vi "LSMcontroller_v61_updatedROIselection.vi"() -> ()   [LabVIEW 2015] (continued)
                            n1350 = call "stoperaseCI.vi"() -> ()  [unwired: 12 in]
                            n1351 = call "stoperaseDO_img.vi"() -> ()  [unwired: 12 in]
                            n1352 = call "stoperaseAO_img.vi"() -> ()  [unwired: 12 in]
                            n1353 = call "stoperaseAI_img.vi"() -> ()  [unwired: 12 in]
                          }
                          frame #7 {
                            w3778 = T22 2 items=["no dialog", "OK message", "continue or stop message", "OK message + warnings", "continue/stop + warnings"] ("type of dialog (OK msg:1)")
                            n1354 = call "displayerrors.vi"() -> ("error IO"=w3779:errorcluster)
                            n1355 = call <vilib>:"General Error Handler.vi"("type of dialog (OK msg:1)"=w3778, "error in (no error)"=w3779) -> ("error out"=w3777:errorcluster)  [unwired: 9 in, 4 out]
                            n1356 = call <vilib>:"Clear Errors.vi"("error in (no error)"=w3777) -> ("error out"=w3776:errorcluster)  [unwired: 5 in, 1 out]
                            n1357 = call "seterrors.vi"("error IO"=w3776) -> ()
                          }
                          frame #8 {
                            w3789 = FALSE ("Value (Signaling)")
                            n1358 = local read "save\ndata"() -> (w3784:bool)
                            n1359 = call "2pparameters.vi"("command"="get") -> ("params out"=w3782:T11)  [unwired: 1 in]
                            n1360 = Unbundle By Name(w3782) -> ("auto OD"=w3780:bool)
                            n1361 = case shown="True" w3784 {
                              tunnel: w3783 -> [_ w3796]
                              frame False {
                              }
                              frame True {
                                n1362 = local read "filename prefix"() -> (w3797:string)
                                n1363 = call "closebinaryfiles.vi"() -> ()  [unwired: 12 in]
                                n1364 = local read "data dir"() -> (w3798:path)
                                n1365 = call "saveparams.vi"("timestamp"=w3796, "filename prefix in"=w3797, "data dir in"=w3798) -> ()  [unwired: 1 in]
                              }
                            }
                            n1366 = case shown="True" w3780 {
                              frame False {
                              }
                              frame True {
                                n1367 = call "configuration.vi"("command"="get") -> ("config out"=w3792:T12)  [unwired: 2 in, 1 out]
                                n1368 = call "2pparameters.vi"("command"="get") -> ("params out"=w3795:T11)  [unwired: 1 in]
                                n1369 = Unbundle By Name(w3792) -> ("point OD"=w3790:u16)
                                n1370 = Unbundle By Name(w3795) -> ("ODfilt"=w3791:u16)
                                n1371 = call "filterwheelcontrol_nothorlabslib.vi"("Current OD filt"=w3790, "New ODfilt"=w3791) -> ()  [unwired: 1 in]
                              }
                            }
                            n1372 = call "reset AO_DO_v3.vi"() -> ()  [unwired: 12 in]
                            n1373 = property on="Start" class="Bool (strict)"("Val(Sgnl)"=w3789) -> ()  [unwired: 2 in, 2 out]
                            n1374 = property on="Start" class="Bool (strict)"("Visible"=TRUE, "DisabledEnum"=T7."Enabled" ("Disabled")) -> ()  [unwired: 2 in, 2 out]
                            n1375 = property on="Stop" class="Bool (strict)"("Val(Sgnl)"=w3789) -> ()  [unwired: 2 in, 2 out]
                            n1376 = property on="Stop" class="Bool (strict)"("Visible"=FALSE, "DisabledEnum"=T7."Disabled" ("Disabled")) -> ()  [unwired: 2 in, 2 out]
                          }
                        }
                      }
                      frame "Line" {
                      }
                      frame "Resonant Ellipse", "freeform contour", "Fill Ellipse" {
                        n1377 = stacked-sequence {
                          seq-local: [w3813 _ _ _ _ _ _ _ _ _ _] -> [_ _ w4658 _ _ w4671 w4738 _ _ w5098 _]
                          seq-local: [w3812 _ _ _ _ _ _ _ _ _ _] -> [_ _ _ _ _ _ _ _ w4785 _ _]
                          seq-local: [w3811 _ _ _ _ _ _ _ _ _ _] -> [_ _ _ _ _ _ _ _ w4784 _ _]
                          seq-local: [w3810 _ _ _ _ _ _ _ _ _ _] -> [_ _ _ _ _ _ _ _ w4787 _ _]
                          seq-local: [w3809 _ _ _ _ _ _ _ _ _ _] -> [_ _ _ _ _ _ _ _ w4783 _ _]
                          seq-local: [w3808 _ _ _ _ _ _ _ _ _ _] -> [_ _ _ _ _ _ _ _ w4782 _ _]
                          seq-local: [w3807 _ _ _ _ _ _ _ _ _ _] -> [_ _ _ _ _ _ _ _ w4786 _ _]
                          seq-local: [w3806 _ _ _ _ _ _ _ _ _ _] -> [_ _ _ _ _ _ _ _ w4781 _ _]
                          seq-local: [w3805 _ _ _ _ _ _ _ _ _ _] -> [_ _ _ _ _ _ _ _ w4780 _ _]
                          seq-local: [w3804 _ _ _ _ _ _ _ _ _ _] -> [_ _ _ _ _ _ _ _ w4775 _ _]
                          seq-local: [w3803 _ _ _ _ _ _ _ _ _ _] -> [_ _ _ _ _ _ _ _ w4774 _ _]
                          seq-local: [w3802 _ _ _ _ _ _ _ _ _ _] -> [_ _ _ _ _ _ _ _ w4779 _ _]
                          seq-local: [w3801 _ _ _ _ _ _ _ _ _ _] -> [_ _ _ _ _ _ _ _ w4778 _ _]
                          seq-local: [w3800 _ _ _ _ _ _ _ _ _ _] -> [_ _ _ _ _ _ _ _ w4777 _ _]
                          seq-local: [w3799 _ _ _ _ _ _ _ _ _ _] -> [_ _ _ _ _ _ _ _ w4776 _ _]
                          frame #0 {
                            n1378 = local read "save\ndata"() -> (w3814:bool)
                            n1379 = Get Date/Time In Seconds() -> (seconds since 1Jan1904=w3815:timestamp)
                            n1380 = case shown="False" w3814 {
                              tunnel: w3815 -> [w3816 w3818]
                              tunnel: [w3816 w3817] -> w3813
                              frame False {
                              }
                              frame True {
                                n1381 = call "createdatafolder.vi"("timestamp in"=w3818) -> ("current data path"=w3819:path, "timestamp out"=w3817:timestamp)
                                n1382 = local write "data dir"(w3819) -> ()
                              }
                            }
                            n1383 = stacked-sequence {
                              tunnel: w3813 -> [w3825 _ _ _ _ _ _ _ _]
                              tunnel: [_ _ _ _ _ _ w3963 _ _] -> w3812
                              tunnel: [_ _ _ _ _ _ w3962 _ _] -> w3811
                              tunnel: [_ _ _ _ _ _ w3961 _ _] -> w3810
                              tunnel: [_ _ _ _ _ _ w3960 _ _] -> w3809
                              tunnel: [_ _ _ _ _ _ w3959 _ _] -> w3808
                              tunnel: [_ _ _ _ _ _ w3958 _ _] -> w3807
                              tunnel: [_ _ _ _ _ _ w3957 _ _] -> w3806
                              tunnel: [_ _ _ _ _ _ w3956 _ _] -> w3805
                              tunnel: [_ _ _ _ _ _ w3955 _ _] -> w3804
                              tunnel: [_ _ _ _ _ _ w3954 _ _] -> w3803
                              tunnel: [_ _ _ _ _ _ w3953 _ _] -> w3802
                              tunnel: [_ _ _ _ _ _ w3952 _ _] -> w3801
                              tunnel: [_ _ _ _ _ _ w3951 _ _] -> w3800
                              tunnel: [_ _ _ _ _ _ w3950 _ _] -> w3799
                              frame #0 {
                                n1384 = local write "graphtab"(T5."timetrace" ("graphtab")) -> ()
                                n1385 = local read "AI channels"() -> (w3829:i32[])
                                n1386 = local read "CI channels"() -> (w3830:i32[])
                                n1387 = property on="Stop" class="Bool (strict)"("Visible"=TRUE, "DisabledEnum"=T7."Enabled" ("Disabled")) -> ()  [unwired: 2 in, 2 out]
                                n1388 = property on="Start" class="Bool (strict)"("Visible"=FALSE, "DisabledEnum"=T7."Disabled and Grayed Out" ("Disabled")) -> ()  [unwired: 2 in, 2 out]
                                n1389 = Format Date/Time String(time format string (%c)="%Y%m%d", seconds (now)=w3825) -> (date/time string=w3824:string)  [unwired: 1 in]
                                n1390 = Format Date/Time String(time format string (%c)="%H%M%S", seconds (now)=w3825) -> (date/time string=w3823:string)  [unwired: 1 in]
                                n1391 = call "2pparameters.vi"("command"="get") -> ("params out"=w3832:T11)  [unwired: 1 in]
                                n1392 = Bundle By Name(cluster=w3832, "aAI"=w3829, "aCI"=w3830, "type"="Timetrace", "date"=w3824, "time"=w3823) -> (w3831:T11)
                                n1393 = call "X-array-databuffer.vi"("command"=enum16{"get", "set", "clear", "append"}."clear") -> ()  [unwired: 3 in, 2 out]
                                n1394 = call "Y-array-databuffer.vi"("command"=enum16{"get", "set", "clear", "append"}."clear") -> ()  [unwired: 3 in, 2 out]
                                n1395 = call "2pparameters.vi"("Params in"=w3831, "command"="set") -> ()  [unwired: 1 out]
                                n1396 = call "CH1-1D-temp.vi"("command"=enum16{"get", "set", "clear", "append"}."clear") -> ()  [unwired: 3 in, 2 out]
                                n1397 = call "CH2-1D-temp.vi"("command"=enum16{"get", "set", "clear", "append"}."clear") -> ()  [unwired: 3 in, 2 out]
                                n1398 = call "allAI-temp.vi"("command"=enum16{"get", "set", "clear", "append"}."clear") -> ()  [unwired: 3 in, 2 out]
                              }
                              frame #1 {
                                n1399 = call "configuration.vi"("command"="get") -> ("config out"=w3849:T12)  [unwired: 2 in, 1 out]
                                n1400 = Unbundle By Name(w3849) -> ("CI names"=w3850:string[], "AI names"=w3851:string[])
                                n1401 = call "2pparameters.vi"("command"="get") -> ("params out"=w3845:T11)  [unwired: 1 in]
                                n1402 = Unbundle By Name(w3845) -> ("aCI"=w3846:i32[], "aAI"=w3847:i32[])
                                n1403 = for {
                                tunnel: w3846 -> [w3861] mode=indexing
                                tunnel: w3850 -> [w3862]
                                tunnel: [w3860] -> w3852 mode=indexing
                                n1404 = Index Array(array=w3862, index=w3861) -> (element=w3860:string)
                                }
                                n1405 = for {
                                tunnel: w3847 -> [w3858] mode=indexing
                                tunnel: w3851 -> [w3859]
                                tunnel: [w3857] -> w3853 mode=indexing
                                n1406 = Index Array(array=w3859, index=w3858) -> (element=w3857:string)
                                }
                                n1407 = Build Array (concatenate)(w3852, w3853) -> (w3843:string[])
                                n1408 = for {
                                tunnel: w3843 -> [w3855] mode=indexing
                                tunnel: [w3854] -> w3842 mode=indexing
                                i -> [w3856]
                                n1409 = Bundle("String"=w3855, w3856) -> (w3854:cluster{"String":string, i32})  [unwired: 1 in]
                                }
                                n1410 = property on="graph1list" class="Ring (strict)"("StringsAndValues[]"=w3842) -> ()  [unwired: 2 in, 2 out]
                                n1411 = property on="graph2list" class="Ring (strict)"("StringsAndValues[]"=w3842) -> ()  [unwired: 2 in, 2 out]
                              }
                              frame #2 {
                                n1412 = call "2pparameters.vi"("command"="get") -> ("params out"=w3865:T11)  [unwired: 1 in]
                                n1413 = Unbundle By Name(w3865) -> ("auto OD"=w3863:bool, "autoshutter"=w3866:bool)
                                n1414 = case shown="True" w3863 {
                                frame False {
                                }
                                frame True {
                                n1415 = call "configuration.vi"("command"="get") -> ("config out"=w3869:T12)  [unwired: 2 in, 1 out]
                                n1416 = Unbundle By Name(w3869) -> ("contour OD"=w3870:u16)
                                n1417 = local read "ODfilt"() -> (w3867:u16)
                                n1418 = call "filterwheelcontrol_nothorlabslib.vi"("Current OD filt"=w3867, "New ODfilt"=w3870) -> ()  [unwired: 1 in]
                                }
                                }
                                n1419 = case shown="True" w3866 {
                                frame False {
                                }
                                frame True {
                                n1420 = call "shuttercontrol.vi"("command"="close") -> ()  [unwired: 1 in, 1 out]
                                }
                                }
                              }
                              frame #3 {
                                n1421 = local read "Vy-min draw"() -> (w3879:dbl)
                                n1422 = local read "Vy-max draw"() -> (w3878:dbl)
                                n1423 = local read "Vx-min draw"() -> (w3881:dbl)
                                n1424 = local read "Vx-max draw"() -> (w3880:dbl)
                                n1425 = local read "xpixels ref"() -> (w3877:i32)
                                n1426 = local read "ypixels ref"() -> (w3876:i32)
                                n1427 = local read "ROI Type"() -> (w3875:u16)
                                n1428 = local read "srateAODOtt"() -> (w3898:dbl)
                                n1429 = local read "# of frames"() -> (w3903:i32)
                                n1430 = local read "refreshtime"() -> (w3895:dbl)
                                n1431 = local read "Pel"() -> (w3874:dbl)
                                n1432 = local read "bin"() -> (w3901:dbl)
                                n1433 = local read "Override AI buffer"() -> (w3872:bool)
                                n1434 = local read "finite samples"() -> (w3910:bool)
                                n1435 = local read "srateAODOtt"() -> (w3897:dbl)
                                n1436 = local read "srateAODOtt"() -> (w3904:dbl)
                                n1437 = local read "continuous"() -> (w3909:bool)
                                n1438 = local read "Angle ref"() -> (w3882:dbl)
                                n1439 = local read "wavdet"() -> (w3911:bool)
                                n1440 = local read "Vx-ref"() -> (w3906:dbl)
                                n1441 = local read "Vy-ref"() -> (w3908:dbl)
                                n1442 = local read "avpp"() -> (w3907:i32)
                                n1443 = call "tt_timeandsamples.vi"("bin"=w3901, "refreshtime"=w3895, "srateAODOtt"=w3898, "tot#ofsamples"=w3903) -> ("refreshrate"=w3899:dbl, "refreshbuffer"=w3900:i32, "timetracecycles"=w3905:i32)  [unwired: 5 in]
                                n1444 = local read "bin"() -> (w3902:dbl)
                                n1445 = call "2pparameters.vi"("command"="get") -> ("params out"=w3914:T11)  [unwired: 1 in]
                                n1446 = Bundle By Name(cluster=w3914, "Drawing Mode"=w3875, "measpoints"=w3903, "tt_cycles"=w3905, "refreshbuffer"=w3900, "refreshrate"=w3899, "Vx-ref"=w3906, "Vy-ref"=w3908, "srate"=w3897, "finite"=w3910, "cont"=w3909, "wavdet"=w3911, "avpp"=w3907, "srateAODO"=w3904, "bufferAI"=w3900, "bin"=w3902, "Angle Img"=w3882, "Vxminref"=w3881, "Vxmaxref"=w3880, "Vyminref"=w3879, "Vymaxref"=w3878, "Xpixels Img"=w3877, "Ypixels Img"=w3876, "Pel"=w3874, "Vz-reset"=0.0, "AIoverride"=w3872) -> (w3912:T11)
                                n1447 = Reciprocal(x=w3899) -> (1/x=w3896:dbl)
                                n1448 = local write "refreshtime"(w3896) -> ()
                                n1449 = call "2pparameters.vi"("Params in"=w3912, "command"="set") -> ()  [unwired: 1 out]
                                n1450 = local read "Voltage Clamp"() -> (w3889:bool)
                                n1451 = local read "Current Clamp"() -> (w3890:bool)
                                n1452 = local read "Vholding (mV)"() -> (w3884:sgl)
                                n1453 = local read "CC_ICgain"() -> (w3888:dbl)
                                n1454 = local read "OCgain"() -> (w3885:sgl)
                                n1455 = local read "holdon"() -> (w3883:bool)
                                n1456 = call "patchparameters.vi"("command"="get") -> ("Params out"=w3892:T14)  [unwired: 1 in]
                                n1457 = Bundle By Name(cluster=w3892, "VC"=w3889, "CC"=w3890, "CC_icg (pA/mv)"=w3888, "VC_icg (mV/mV)"=10.0, "OCG (mV/pA)"=w3885, "OVG (mV/mV)"=0.1, "Vhold (mV)"=w3884, "holdon"=w3883) -> (w3891:T14)
                                n1458 = call "patchparameters.vi"("Params in"=w3891, "command"="set") -> ()  [unwired: 1 out]
                              }
                              frame #4 {
                                n1459 = call "2pparameters.vi"("command"="get") -> ("params out"=w3930:T11)  [unwired: 1 in]
                                n1460 = Unbundle By Name(w3930) -> ("srateAODO"=w3931:sgl, "Angle Img"=w3932:dbl, "Angle draw"=w3933:dbl, "Vxmaxref"=w3934:dbl, "Vxminref"=w3935:dbl, "Xpixels Img"=w3936:i32, "Ypixels Img"=w3937:i32, "Vymaxref"=w3938:dbl, "Vxminref"=w3939:dbl, "Drawing Mode"=w3940:u16, "Pel"=w3941:sgl)
                                n1461 = Add(x=w3932, y=w3933) -> (x+y=w3916:dbl)
                                n1462 = call "ROI-databuffer.vi"("command"=enum16{"get", "set", "clear", "append"}."get") -> ("array out"=w3924:cluster{"x":sgl, "y":sgl}[])  [unwired: 4 in]
                                n1463 = call "ScanningWaveform_v4.vi"("Vy-min"=w3939, "Vy-max"=w3938, "yPixels/tPixels"=w3937, "xPixels/rPixels"=w3936, "Vx-min"=w3935, "Vx-max"=w3934, "Drawing Mode"=w3940, "Angle"=w3916, "AOrate"=w3931, "Points"=w3924, "points in ellipse"=w3941) -> ("numPixels"=w3917:dbl, "Y-WaveArray"=w3918:dbl[], "P"=w3923:dbl, "X-WaveArray"=w3919:dbl[])  [unwired: 5 in]
                                n1464 = call "Y-array-databuffer.vi"("array in"=w3918, "command"=enum16{"get", "set", "clear", "append"}."set") -> ()  [unwired: 2 in, 2 out]
                                n1465 = call "X-array-databuffer.vi"("array in"=w3919, "command"=enum16{"get", "set", "clear", "append"}."set") -> ()  [unwired: 2 in, 2 out]
                                n1466 = call "2pparameters.vi"("command"="get") -> ("params out"=w3928:T11)  [unwired: 1 in]
                                n1467 = Bundle By Name(cluster=w3928, "P"=w3923, "sAOxy"=w3917, "Pel"=w3917) -> (w3920:T11)
                                n1468 = call "2pparameters.vi"("Params in"=w3920, "command"="set") -> ()  [unwired: 1 out]
                              }
                              frame #5 {
                                n1469 = call "X-array-databuffer.vi"("command"=enum16{"get", "set", "clear", "append"}."get") -> ("array out"=w3944:dbl[])  [unwired: 3 in, 1 out]
                                n1470 = call "Y-array-databuffer.vi"("command"=enum16{"get", "set", "clear", "append"}."get") -> ("array out"=w3947:dbl[])  [unwired: 3 in, 1 out]
                                n1471 = Index Array(array=w3944, index=0) -> (element=w3943:dbl)
                                n1472 = Index Array(array=w3947, index=0) -> (element=w3942:dbl)
                                n1473 = call "setposition.vi"("Vy"=w3942, "Vx"=w3943) -> ()  [unwired: 1 in]
                              }
                              frame #6 {
                                # "rem2Ps"
                                # "A2Ps"
                                # "Al"
                                # "Rl"
                                n1474 = stacked-sequence {
                                seq-local: [w3968 _ _ _ _ _ _ _ _ _ _] -> [_ w4080 _ w4141 _ w4227 _ _ _ _ _]
                                seq-local: [w3969 _ _ _ _ _ _ _ _ _ _] -> [_ w4081 w4091 _ w4196 _ _ _ _ _ _]
                                seq-local: [_ _ w4090 _ _ _ _ _ _ _ _] -> [_ _ _ _ w4190 _ _ _ _ _ _]
                                seq-local: [_ _ _ w4140 _ _ _ _ _ _ _] -> [_ _ _ _ _ w4226 _ _ _ _ _]
                                seq-local: [w3965 _ _ _ _ _ _ _ _ _ _] -> [_ w4077 _ _ _ _ _ _ w4412 w4480 _]
                                seq-local: [w3964 _ _ _ _ _ _ _ _ _ _] -> [_ w4076 _ _ _ _ _ _ w4413 w4481 _]
                                seq-local: [w3971 _ _ _ _ _ _ _ _ _ _] -> [_ _ _ _ _ _ w4265 _ w4411 w4479 _]
                                seq-local: [w3967 _ _ _ _ _ _ _ _ _ _] -> [_ w4075 _ _ _ _ w4264 w4332 _ _ _]
                                seq-local: [w3966 _ _ _ _ _ _ _ _ _ _] -> [_ w4074 _ _ _ _ w4263 w4331 _ _ _]
                                seq-local: [w3970 _ _ _ _ _ _ _ _ _ _] -> [_ _ _ _ _ _ w4262 w4330 _ _ _]
                                tunnel: [_ _ w4089 _ _ _ _ _ _ _ _] -> w3962
                                tunnel: [_ _ w4088 _ _ _ _ _ _ _ _] -> w3963
                                tunnel: [w3969 _ _ _ _ _ _ _ _ _ _] -> w3961
                                tunnel: [w3968 _ _ _ _ _ _ _ _ _ _] -> w3958
                                tunnel: [_ _ _ w4139 _ _ _ _ _ _ _] -> w3959
                                tunnel: [_ _ _ w4138 _ _ _ _ _ _ _] -> w3960
                                tunnel: [w3967 _ _ _ _ _ _ _ _ _ _] -> w3953
                                tunnel: [w3966 _ _ _ _ _ _ _ _ _ _] -> w3952
                                tunnel: [_ _ _ _ _ _ w4261 _ _ _ _] -> w3951
                                tunnel: [_ _ _ _ _ _ _ w4329 _ _ _] -> w3950
                                tunnel: [w3965 _ _ _ _ _ _ _ _ _ _] -> w3954
                                tunnel: [w3964 _ _ _ _ _ _ _ _ _ _] -> w3955
                                tunnel: [_ _ _ _ _ _ _ _ w4410 _ _] -> w3956
                                tunnel: [_ _ _ _ _ _ _ _ _ w4478 _] -> w3957
                                frame #0 {
                                # "for a next version, give ome thought to\nthe possibilit of intermittently updating the\nwaveforms. it will have to be a calculation\nbased on speed of CPU and program on the one hand\nand length of measurement on the other. but then it should be possible, in principle, to \nupdate the waveform on the fly and that way cut up a longer measurement in smaller parts."
                                n1475 = stacked-sequence {
                                tunnel: [w3972 _ _ _] -> w3969
                                tunnel: [_ w3984 _ _] -> w3968
                                tunnel: [_ _ _ w4041] -> w3964
                                tunnel: [_ _ _ w4040] -> w3965
                                tunnel: [_ _ _ w4039] -> w3971
                                tunnel: [_ _ w3999 _] -> w3967
                                tunnel: [_ _ w3998 _] -> w3966
                                tunnel: [_ _ w3997 _] -> w3970
                                frame #0 {
                                n1476 = call "configuration.vi"("command"="get") -> ("config out"=w3974:T12)  [unwired: 2 in, 1 out]
                                n1477 = Unbundle By Name(w3974) -> ("Voltage to Xgalvo"=w3973:i32)
                                n1478 = call "2pparameters.vi"("command"="get") -> ("params out"=w3978:T11)  [unwired: 1 in]
                                n1479 = in-place {
                                in-place-border: w3973 -> [w3983]
                                in-place-border: [w3980] -> w3972
                                n1480 = in-place-cluster #23(w3978) -> ("aAO"=w3982:u32[])
                                n1481 = call "add channel to active arrayv2.vi"("line array in"=w3982, "line to add"=w3983) -> ("line array out"=w3981:u32[], "addition"=w3980:bool)  [unwired: 1 out]
                                n1482 = in-place-cluster #23("aAO"=w3981) -> (w3976:T11)
                                }
                                n1483 = call "2pparameters.vi"("Params in"=w3976, "command"="set") -> ()  [unwired: 1 out]
                                }
                                frame #1 {
                                n1484 = call "configuration.vi"("command"="get") -> ("config out"=w3986:T12)  [unwired: 2 in, 1 out]
                                n1485 = Unbundle By Name(w3986) -> ("Voltage to Ygalvo"=w3985:i32)
                                n1486 = call "2pparameters.vi"("command"="get") -> ("params out"=w3990:T11)  [unwired: 1 in]
                                n1487 = in-place {
                                in-place-border: w3985 -> [w3995]
                                in-place-border: [w3992] -> w3984
                                n1488 = in-place-cluster #24(w3990) -> ("aAO"=w3994:u32[])
                                n1489 = call "add channel to active arrayv2.vi"("line array in"=w3994, "line to add"=w3995) -> ("line array out"=w3993:u32[], "addition"=w3992:bool)  [unwired: 1 out]
                                n1490 = in-place-cluster #24("aAO"=w3993) -> (w3988:T11)
                                }
                                n1491 = call "2pparameters.vi"("Params in"=w3988, "command"="set") -> ()  [unwired: 1 out]
                                }
                                frame #2 {
                                n1492 = call "2pparameters.vi"("command"="get") -> ("params out"=w4001:T11)  [unwired: 1 in]
                                n1493 = Unbundle By Name(w4001) -> ("autoshutter"=w4000:bool, "wavdet"=w3996:bool)
                                n1494 = case shown="False" w4000 {
                                tunnel: [w4006 w4026] -> w3999
                                tunnel: [w4005 FALSE ("removal")] -> w3998
                                tunnel: [w4004 w4024] -> w3997
                                tunnel: w3996 -> [w4003 _]
                                frame False {
                                n1495 = case shown="False" w4003 {
                                tunnel: [FALSE ("addition") FALSE ("addition")] -> w4006
                                tunnel: [w4008 FALSE ("removal")] -> w4005
                                tunnel: [w4007 _] -> w4004
                                frame False {
                                n1496 = call "configuration.vi"("command"="get") -> ("config out"=w4014:T12)  [unwired: 2 in, 1 out]
                                n1497 = Unbundle By Name(w4014) -> ("2P shutter"=w4011:i32)
                                n1498 = call "2pparameters.vi"("command"="get") -> ("params out"=w4012:T11)  [unwired: 1 in]
                                n1499 = in-place {
                                in-place-border: w4011 -> [w4021]
                                in-place-border: [w4018] -> w4008
                                in-place-border: [w4017] -> w4007
                                n1500 = in-place-cluster #25(w4012) -> ("aDO"=w4020:u32[])
                                n1501 = call "remove channel from active arrayv2.vi"("line array in"=w4020, "line to remove"=w4021) -> ("line array out"=w4019:u32[], "removal"=w4018:bool, "index"=w4017:i32)
                                n1502 = in-place-cluster #25("aDO"=w4019) -> (w4009:T11)
                                }
                                n1503 = call "2pparameters.vi"("Params in"=w4009, "command"="set") -> ()  [unwired: 1 out]
                                }
                                frame True {
                                }
                                }
                                }
                                frame True {
                                n1504 = call "configuration.vi"("command"="get") -> ("config out"=w4028:T12)  [unwired: 2 in, 1 out]
                                n1505 = call "2pparameters.vi"("command"="get") -> ("params out"=w4032:T11)  [unwired: 1 in]
                                n1506 = Unbundle By Name(w4028) -> ("2P shutter"=w4027:i32)
                                n1507 = in-place {
                                in-place-border: w4027 -> [w4038]
                                in-place-border: [w4035] -> w4026
                                in-place-border: [w4034] -> w4024
                                n1508 = in-place-cluster #26(w4032) -> ("aDO"=w4037:u32[])
                                n1509 = call "add channel to active arrayv2.vi"("line array in"=w4037, "line to add"=w4038) -> ("line array out"=w4036:u32[], "addition"=w4035:bool, "index"=w4034:i32)
                                n1510 = in-place-cluster #26("aDO"=w4036) -> (w4030:T11)
                                }
                                n1511 = call "2pparameters.vi"("Params in"=w4030, "command"="set") -> ()  [unwired: 1 out]
                                }
                                }
                                }
                                frame #3 {
                                n1512 = local read "Measurement"() -> (w4042:T4)
                                n1513 = To Unsigned Long Integer(number=w4042) -> (unsigned 32bit integer=w4043:u32)
                                n1514 = case shown="5..7" w4043 {
                                tunnel: [FALSE ("addition") w4061] -> w4041
                                tunnel: [w4046 FALSE ("removal")] -> w4040
                                tunnel: [w4044 w4059] -> w4039
                                frame 0..4, Default {
                                n1515 = call "configuration.vi"("command"="get") -> ("config out"=w4052:T12)  [unwired: 2 in, 1 out]
                                n1516 = Unbundle By Name(w4052) -> ("LT timestamp"=w4049:u32)
                                n1517 = call "2pparameters.vi"("command"="get") -> ("params out"=w4050:T11)  [unwired: 1 in]
                                n1518 = in-place {
                                in-place-border: w4049 -> [w4058]
                                in-place-border: [w4055] -> w4046
                                in-place-border: [w4054] -> w4044
                                n1519 = in-place-cluster #27(w4050) -> ("aDO"=w4057:u32[])
                                n1520 = call "remove channel from active arrayv2.vi"("line array in"=w4057, "line to remove"=w4058) -> ("line array out"=w4056:u32[], "removal"=w4055:bool, "index"=w4054:i32)
                                n1521 = in-place-cluster #27("aDO"=w4056) -> (w4047:T11)
                                }
                                n1522 = call "2pparameters.vi"("Params in"=w4047, "command"="set") -> ()  [unwired: 1 out]
                                }
                                frame 5..7 {
                                n1523 = call "configuration.vi"("command"="get") -> ("config out"=w4067:T12)  [unwired: 2 in, 1 out]
                                n1524 = Unbundle By Name(w4067) -> ("LT timestamp"=w4064:u32)
                                n1525 = call "2pparameters.vi"("command"="get") -> ("params out"=w4065:T11)  [unwired: 1 in]
                                n1526 = in-place {
                                in-place-border: w4064 -> [w4073]
                                in-place-border: [w4070] -> w4061
                                in-place-border: [w4069] -> w4059
                                n1527 = in-place-cluster #28(w4065) -> ("aDO"=w4072:u32[])
                                n1528 = call "add channel to active arrayv2.vi"("line array in"=w4072, "line to add"=w4073) -> ("line array out"=w4071:u32[], "addition"=w4070:bool, "index"=w4069:i32)
                                n1529 = in-place-cluster #28("aDO"=w4071) -> (w4062:T11)
                                }
                                n1530 = call "2pparameters.vi"("Params in"=w4062, "command"="set") -> ()  [unwired: 1 out]
                                }
                                }
                                }
                                }
                                }
                                frame #1 {
                                n1531 = Or(x=w4080, y=w4081) -> (x .or. y?=w4079:bool)
                                n1532 = case shown="True" w4079 {
                                frame False {
                                }
                                frame True {
                                # "update GUI"
                                n1533 = call "Used AO lines.vi"() -> ("used AO names"=w4085:string[], "used AO lines"=w4087:tag[])  [unwired: 2 in]
                                n1534 = control-ref of="Analog Lines Plot"() -> (w4086:refnum<vi>)
                                n1535 = local write "Analog Used Lines"(w4087) -> ()
                                n1536 = local write "Analog Used Names"(w4085) -> ()
                                n1537 = call "prepAOWaveplot.vi"("WaveformGraph in"=w4086, "Analog Used Names"=w4085) -> ()  [unwired: 1 in]
                                }
                                }
                                n1538 = Compound Arithmetic op=OR(w4077, w4076, w4075, w4074) -> (w4078:bool)
                                n1539 = case shown="True" w4078 {
                                frame False {
                                }
                                frame True {
                                n1540 = control-ref of="Digital Lines Plot"() -> (w4082:refnum<vi>)
                                n1541 = call "Used DO lines.vi"() -> ("used DO names"=w4083:string[], "used DO lines"=w4084:tag[])  [unwired: 2 in]
                                n1542 = local write "Digital Used Lines"(w4084) -> ()
                                n1543 = local write "Digital Used Names"(w4083) -> ()
                                n1544 = call "prepDOWaveplot.vi"("DigitalGraph in"=w4082, "used DO names"=w4083) -> ()  [unwired: 1 in]
                                }
                                }
                                }
                                frame #2 {
                                n1545 = case shown="False" w4091 {
                                tunnel: [w4094 w4120] -> w4090
                                tunnel: [w4093 w4118] -> w4089
                                tunnel: [w4092 _] -> w4088
                                frame False {
                                n1546 = stacked-sequence {
                                seq-local: [w4096 _] -> [_ w4111]
                                tunnel: [w4096 _] -> w4094
                                tunnel: [w4099 _] -> w4093
                                tunnel: [w4095 _] -> w4092
                                frame #0 {
                                n1547 = call "configuration.vi"("command"="get") -> ("config out"=w4107:T12)  [unwired: 2 in, 1 out]
                                n1548 = call "waveformparamsv2.vi"("command"="get") -> ("Params out"=w4101:T15)  [unwired: 4 in, 2 out]
                                n1549 = Unbundle By Name(w4107) -> ("Voltage to Xgalvo"=w4108:i32)
                                n1550 = call "2pparameters.vi"("command"="get") -> ("params out"=w4104:T11)  [unwired: 1 in]
                                n1551 = Unbundle By Name(w4101) -> ("AO parameters"=w4100:T16)
                                n1552 = Unbundle By Name(w4104) -> ("aAO"=w4105:u32[])
                                n1553 = call "waveformsAObuffer.vi"("command"="get") -> ("AO wf out"=w4097:waveform(dbl)[])  [unwired: 1 in]
                                n1554 = Search 1D Array(1D array=w4105, element=w4108) -> (index of element=w4096:i32)  [unwired: 1 in]
                                n1555 = Index Array(array=w4097, index=w4096) -> (element=w4095:waveform(dbl))
                                n1556 = Index Array(array=w4100, index=w4096) -> (element=w4099:T17)
                                }
                                frame #1 {
                                w4112 = 0.0 ("Step size (V)")
                                n1557 = local read "Meastab"() -> (w4110:enum32{"X-Y Image", "Linescan", "Timetrace"})
                                n1558 = case shown="\"X-Y Image\", Default" w4110 {
                                tunnel: [w4114 w4115] -> w4109
                                frame "X-Y Image", Default {
                                n1559 = local read "Sampling rate"() -> (w4114:dbl)
                                }
                                frame "Timetrace" {
                                n1560 = local read "srateAODOtt"() -> (w4115:dbl)
                                }
                                }
                                n1561 = call "replace AO XYwfparam.vi"("Baseline (V)"=w4112, "Start amplitude (V)"=w4112, "Cycles"=w4112, "Repeats"=w4112, "index of AO wave"=w4111, "Step size (V)"=w4112, "DC (%)"=w4112, "Sampling frequency (Hz)"=w4109, "Period (ms)"=w4112, "Cycle length (s)"=w4112, "Pulses"=w4112, "padding value"=w4112, "Matlab wave name"=path "xwave") -> ()  [unwired: 3 in]
                                }
                                }
                                }
                                frame True {
                                w4119 = 0.0 ("Repeats")
                                n1562 = local read "Meastab"() -> (w4117:enum32{"X-Y Image", "Linescan", "Timetrace"})
                                n1563 = case shown="\"X-Y Image\", Default" w4117 {
                                tunnel: [w4136 w4137] -> w4116
                                frame "X-Y Image", Default {
                                n1564 = local read "Sampling rate"() -> (w4136:dbl)
                                }
                                frame "Timetrace" {
                                n1565 = local read "srateAODOtt"() -> (w4137:dbl)
                                }
                                }
                                n1566 = call "2pparameters.vi"("command"="get") -> ("params out"=w4122:T11)  [unwired: 1 in]
                                n1567 = call "configuration.vi"("command"="get") -> ("config out"=w4125:T12)  [unwired: 2 in, 1 out]
                                n1568 = call "waveformparamsv2.vi"("command"="get") -> ("Params out"=w4133:T15)  [unwired: 4 in, 2 out]
                                n1569 = Unbundle By Name(w4125) -> ("Voltage to Xgalvo"=w4126:i32)
                                n1570 = Unbundle By Name(w4133) -> ("AO parameters"=w4130:T16)
                                n1571 = Unbundle By Name(w4122) -> ("aAO"=w4123:u32[])
                                n1572 = Search 1D Array(1D array=w4123, element=w4126) -> (index of element=w4120:i32)  [unwired: 1 in]
                                n1573 = Index Array(array=w4130, index=0) -> (element=w4131:T17)
                                n1574 = Bundle By Name(cluster=w4131, "AOtab"=-1.0 ("Repeats"), "Repeats"=w4119, "Cycles"=w4119, "Start amplitude (V)"=w4119, "Baseline (V)"=w4119, "Step size (V)"=w4119, "DC (%)"=w4119, "Sampling frequency (Hz)"=w4116, "Period (ms)"=w4119, "Offset (V)"=w4119, "Amplitude (V)"=w4119, "Frequency"=w4119, "Tri Repeats"=w4119, "phase shift (ms)"=w4119, "Pulses"=w4119, "Matlab wave file"=path "xwave", "padding value"=w4119) -> (w4118:T17)
                                n1575 = Build Array(w4118) -> (w4128:T16)
                                n1576 = call "waveformparamsv2.vi"("command"="add AO", "add AO"=w4128) -> ()  [unwired: 3 in, 3 out]
                                }
                                }
                                }
                                frame #3 {
                                n1577 = case shown="True" w4141 {
                                tunnel: [w4144 w4170] -> w4140
                                tunnel: [w4143 w4168] -> w4139
                                tunnel: [w4142 _] -> w4138
                                frame False {
                                n1578 = stacked-sequence {
                                seq-local: [w4146 _] -> [_ w4161]
                                tunnel: [w4146 _] -> w4144
                                tunnel: [w4149 _] -> w4143
                                tunnel: [w4145 _] -> w4142
                                frame #0 {
                                n1579 = call "configuration.vi"("command"="get") -> ("config out"=w4157:T12)  [unwired: 2 in, 1 out]
                                n1580 = call "waveformparamsv2.vi"("command"="get") -> ("Params out"=w4151:T15)  [unwired: 4 in, 2 out]
                                n1581 = Unbundle By Name(w4157) -> ("Voltage to Ygalvo"=w4158:i32)
                                n1582 = call "2pparameters.vi"("command"="get") -> ("params out"=w4154:T11)  [unwired: 1 in]
                                n1583 = Unbundle By Name(w4151) -> ("AO parameters"=w4150:T16)
                                n1584 = Unbundle By Name(w4154) -> ("aAO"=w4155:u32[])
                                n1585 = call "waveformsAObuffer.vi"("command"="get") -> ("AO wf out"=w4147:waveform(dbl)[])  [unwired: 1 in]
                                n1586 = Search 1D Array(1D array=w4155, element=w4158) -> (index of element=w4146:i32)  [unwired: 1 in]
                                n1587 = Index Array(array=w4147, index=w4146) -> (element=w4145:waveform(dbl))
                                n1588 = Index Array(array=w4150, index=w4146) -> (element=w4149:T17)
                                }
                                frame #1 {
                                w4162 = 0.0 ("Step size (V)")
                                n1589 = local read "Meastab"() -> (w4160:enum32{"X-Y Image", "Linescan", "Timetrace"})
                                n1590 = case shown="\"X-Y Image\", Default" w4160 {
                                tunnel: [w4164 w4165] -> w4159
                                frame "X-Y Image", Default {
                                n1591 = local read "Sampling rate"() -> (w4164:dbl)
                                }
                                frame "Timetrace" {
                                n1592 = local read "srateAODOtt"() -> (w4165:dbl)
                                }
                                }
                                n1593 = call "replace AO XYwfparam.vi"("Baseline (V)"=w4162, "Start amplitude (V)"=w4162, "Cycles"=w4162, "Repeats"=w4162, "index of AO wave"=w4161, "Step size (V)"=w4162, "DC (%)"=w4162, "Sampling frequency (Hz)"=w4159, "Period (ms)"=w4162, "Cycle length (s)"=w4162, "Pulses"=w4162, "padding value"=w4162, "Matlab wave name"=path "ywave") -> ()  [unwired: 3 in]
                                }
                                }
                                }
                                frame True {
                                w4169 = 0.0 ("Repeats")
                                n1594 = local read "Meastab"() -> (w4167:enum32{"X-Y Image", "Linescan", "Timetrace"})
                                n1595 = case shown="\"X-Y Image\", Default" w4167 {
                                tunnel: [w4186 w4187] -> w4166
                                frame "X-Y Image", Default {
                                n1596 = local read "Sampling rate"() -> (w4186:dbl)
                                }
                                frame "Timetrace" {
                                n1597 = local read "srateAODOtt"() -> (w4187:dbl)
                                }
                                }
                                n1598 = call "2pparameters.vi"("command"="get") -> ("params out"=w4172:T11)  [unwired: 1 in]
                                n1599 = call "configuration.vi"("command"="get") -> ("config out"=w4175:T12)  [unwired: 2 in, 1 out]
                                n1600 = call "waveformparamsv2.vi"("command"="get") -> ("Params out"=w4184:T15)  [unwired: 4 in, 2 out]
                                n1601 = Unbundle By Name(w4175) -> ("Voltage to Ygalvo"=w4176:i32)
                                n1602 = Unbundle By Name(w4184) -> ("AO parameters"=w4181:T16)
                                n1603 = Unbundle By Name(w4172) -> ("aAO"=w4173:u32[])
                                n1604 = Search 1D Array(1D array=w4173, element=w4176) -> (index of element=w4170:i32)  [unwired: 1 in]
                                n1605 = Index Array(array=w4181, index=0) -> (element=w4182:T17)
                                n1606 = Bundle By Name(cluster=w4182, "AOtab"=-1.0 ("Repeats"), "Repeats"=w4169, "Cycles"=w4169, "Start amplitude (V)"=w4169, "Baseline (V)"=w4169, "Step size (V)"=w4169, "DC (%)"=w4169, "Sampling frequency (Hz)"=w4166, "Period (ms)"=w4169, "Offset (V)"=w4169, "Amplitude (V)"=w4169, "Frequency"=w4169, "Tri Repeats"=w4169, "phase shift (ms)"=w4169, "Pulses"=w4169, "Matlab wave file"=path "ywave", "padding value"=w4169) -> (w4168:T17)
                                n1607 = Build Array(w4168) -> (w4179:T16)
                                n1608 = call "waveformparamsv2.vi"("command"="add AO", "add AO"=w4179) -> ()  [unwired: 3 in, 3 out]
                                }
                                }
                                }
                                frame #4 {
                                n1609 = call "2pparameters.vi"("command"="get") -> ("params out"=w4193:T11)  [unwired: 1 in]
                                n1610 = Unbundle By Name(w4193) -> ("wavdet"=w4192:bool, "Pel"=w4189:sgl, "refwfsize"=w4188:dbl, "srateAODO"=w4191:sgl)
                                n1611 = case shown="True" w4192 {
                                tunnel: [w4197 w4207] -> w4195
                                tunnel: w4191 -> [w4198 w4209]
                                tunnel: w4189 -> [_ w4205]
                                tunnel: w4188 -> [_ w4204]
                                frame False {
                                n1612 = call "X-array-databuffer.vi"("command"=enum16{"get", "set", "clear", "append"}."get") -> ("array out"=w4201:dbl[])  [unwired: 3 in, 1 out]
                                n1613 = Reciprocal(x=w4198) -> (1/x=w4199:sgl)
                                n1614 = Bundle By Name("Y"=w4201, "dt"=w4199) -> (w4197:waveform(dbl))  [unwired: 1 in]
                                }
                                frame True {
                                n1615 = To Double Precision Float(number=w4205) -> (double precision float=w4206:dbl)
                                n1616 = Divide(x=w4204, y=w4206) -> (x/y=w4203:dbl)
                                n1617 = Round Toward +Infinity(x=w4203) -> (ceil(x): smallest int >= x=w4202:dbl)
                                n1618 = call "X-array-databuffer.vi"("command"=enum16{"get", "set", "clear", "append"}."get") -> ("array out"=w4211:dbl[])  [unwired: 3 in, 1 out]
                                n1619 = Reciprocal(x=w4209) -> (1/x=w4210:sgl)
                                n1620 = for {
                                N: w4202 -> [_]
                                tunnel: w4211 -> [w4213]
                                tunnel: [w4213] -> w4208 mode=concatenating
                                }
                                n1621 = Bundle By Name("Y"=w4208, "dt"=w4210) -> (w4207:waveform(dbl))  [unwired: 1 in]
                                }
                                }
                                n1622 = case shown="True" w4196 {
                                tunnel: w4195 -> [w4215 w4221]
                                tunnel: w4190 -> [w4216 _]
                                frame False {
                                n1623 = call "waveformsAObuffer.vi"("command"="get") -> ("AO wf out"=w4219:waveform(dbl)[])  [unwired: 1 in]
                                n1624 = property on="refwf" class="Ring (strict)" props=["RingText", "Text"]() -> ()  [unwired: 2 in, 3 out]
                                n1625 = Replace Array Subset(array=w4219, new element=w4215, index=w4216) -> (w4214:waveform(dbl)[])
                                n1626 = call "waveformsAObuffer.vi"("AO wf in"=w4214, "command"="set") -> ()  [unwired: 1 out]
                                }
                                frame True {
                                n1627 = call "waveformsAObuffer.vi"("command"="get") -> ("AO wf out"=w4223:waveform(dbl)[])  [unwired: 1 in]
                                n1628 = Build Array (concatenate)(w4223, w4221) -> (w4220:waveform(dbl)[])
                                n1629 = call "waveformsAObuffer.vi"("AO wf in"=w4220, "command"="set") -> ()  [unwired: 1 out]
                                }
                                }
                                }
                                frame #5 {
                                n1630 = call "2pparameters.vi"("command"="get") -> ("params out"=w4235:T11)  [unwired: 1 in]
                                n1631 = Unbundle By Name(w4235) -> ("wavdet"=w4234:bool, "Pel"=w4232:sgl, "refwfsize"=w4233:dbl, "srateAODO"=w4228:sgl)
                                n1632 = To Double Precision Float(number=w4232) -> (double precision float=w4231:dbl)
                                n1633 = Divide(x=w4233, y=w4231) -> (x/y=w4230:dbl)
                                n1634 = Round Toward +Infinity(x=w4230) -> (ceil(x): smallest int >= x=w4229:dbl)
                                n1635 = case shown="True" w4234 {
                                tunnel: [w4239 w4245] -> w4225
                                tunnel: w4229 -> [_ w4242]
                                tunnel: w4228 -> [w4240 w4247]
                                frame False {
                                n1636 = call "Y-array-databuffer.vi"("command"=enum16{"get", "set", "clear", "append"}."get") -> ("array out"=w4237:dbl[])  [unwired: 3 in, 1 out]
                                n1637 = Reciprocal(x=w4240) -> (1/x=w4241:sgl)
                                n1638 = Bundle By Name("Y"=w4237, "dt"=w4241) -> (w4239:waveform(dbl))  [unwired: 1 in]
                                }
                                frame True {
                                n1639 = call "Y-array-databuffer.vi"("command"=enum16{"get", "set", "clear", "append"}."get") -> ("array out"=w4243:dbl[])  [unwired: 3 in, 1 out]
                                n1640 = Reciprocal(x=w4247) -> (1/x=w4248:sgl)
                                n1641 = for {
                                N: w4242 -> [_]
                                tunnel: w4243 -> [w4249]
                                tunnel: [w4249] -> w4246 mode=concatenating
                                }
                                n1642 = Bundle By Name("Y"=w4246, "dt"=w4248) -> (w4245:waveform(dbl))  [unwired: 1 in]
                                }
                                }
                                n1643 = case shown="False" w4227 {
                                tunnel: w4225 -> [w4252 w4257]
                                tunnel: w4226 -> [w4253 _]
                                frame False {
                                n1644 = call "waveformsAObuffer.vi"("command"="get") -> ("AO wf out"=w4255:waveform(dbl)[])  [unwired: 1 in]
                                n1645 = Replace Array Subset(array=w4255, new element=w4252, index=w4253) -> (w4250:waveform(dbl)[])
                                n1646 = call "waveformsAObuffer.vi"("AO wf in"=w4250, "command"="set") -> ()  [unwired: 1 out]
                                }
                                frame True {
                                n1647 = call "waveformsAObuffer.vi"("command"="get") -> ("AO wf out"=w4259:waveform(dbl)[])  [unwired: 1 in]
                                n1648 = Build Array (concatenate)(w4259, w4257) -> (w4256:waveform(dbl)[])
                                n1649 = call "waveformsAObuffer.vi"("AO wf in"=w4256, "command"="set") -> ()  [unwired: 1 out]
                                }
                                }
                                }
                                frame #6 {
                                n1650 = Build Array(w4264, w4263) -> (w4267:bool[])
                                n1651 = Boolean Array To Number(Boolean array=w4267) -> (number=w4266:u32)
                                n1652 = case shown="1" w4266 {
                                tunnel: w4265 -> [_ _ _ _]
                                tunnel: w4262 -> [_ w4290 _ w4303]
                                tunnel: [_ w4289 _ w4300] -> w4261
                                frame 1 {
                                w4277 = 0.0 ("DOtab")
                                n1653 = call "2pparameters.vi"("command"="get") -> ("params out"=w4274:T11)  [unwired: 1 in]
                                n1654 = call "waveformparamsv2.vi"("command"="get") -> ("Params out"=w4285:T15)  [unwired: 4 in, 2 out]
                                n1655 = Unbundle By Name(w4285) -> ("DO parameters"=w4283:T18)
                                n1656 = Unbundle By Name(w4274) -> ("srate"=w4270:sgl, "Pel"=w4273:sgl)
                                n1657 = To Double Precision Float(number=w4270) -> (double precision float=w4268:dbl)
                                n1658 = To Double Precision Float(number=w4270) -> (double precision float=w4269:dbl)
                                n1659 = To Double Precision Float(number=w4273) -> (double precision float=w4272:dbl)
                                n1660 = Divide(x=w4269, y=w4272) -> (x/y=w4271:dbl)
                                n1661 = Index Array(array=w4283, index=0) -> (element=w4282:T19)
                                n1662 = Bundle By Name(cluster=w4282, "Digital DC (%)"=100.0, "Digital phase"=w4277, "Digital Freq (Hz)"=w4271, "Sampling frequency (Hz)"=w4268, "Digital time offset (s)"=w4277, "padding value"=0.0, "matlab wave file"=path "2Pshutter", "DOtab"=0.0) -> (w4280:T19)
                                n1663 = Build Array(w4280) -> (w4279:T18)
                                n1664 = call "waveformparamsv2.vi"("command"="add DO", "add DO"=w4279) -> ()  [unwired: 3 in, 3 out]
                                }
                                frame 2 {
                                n1665 = call "waveformparamsv2.vi"("command"="get") -> ("Params out"=w4292:T15)  [unwired: 4 in, 2 out]
                                n1666 = in-place {
                                in-place-border: w4290 -> [w4296]
                                in-place-border: [w4295] -> w4289
                                n1667 = in-place-cluster #29(w4292) -> ("DO parameters"=w4298:T18)
                                n1668 = Delete From Array(array=w4298, length=1, index=w4296) -> (deleted portion=w4295:T18, array with subset deleted=w4297:T18)
                                n1669 = in-place-cluster #29("DO parameters"=w4297) -> (w4291:T15)
                                }
                                n1670 = call "waveformparamsv2.vi"("command"="set", "Params in"=w4291) -> ()  [unwired: 3 in, 3 out]
                                }
                                frame 3, Default {
                                }
                                frame 0 {
                                n1671 = call "2pparameters.vi"("command"="get") -> ("params out"=w4305:T11)  [unwired: 1 in]
                                n1672 = Unbundle By Name(w4305) -> ("wavdet"=w4302:bool, "autoshutter"=w4304:bool)
                                n1673 = case shown="True" w4304 {
                                tunnel: w4303 -> [_ w4309]
                                tunnel: w4302 -> [_ w4308]
                                tunnel: [_ w4307] -> w4301
                                frame False {
                                }
                                frame True {
                                n1674 = case shown="False" w4308 {
                                tunnel: w4309 -> [w4311 _]
                                tunnel: [w4310 _] -> w4307
                                frame False {
                                n1675 = stacked-sequence {
                                tunnel: w4311 -> [w4313 w4327]
                                tunnel: [w4312 _] -> w4310
                                frame #0 {
                                n1676 = call "waveformparamsv2.vi"("command"="get") -> ("Params out"=w4315:T15)  [unwired: 4 in, 2 out]
                                n1677 = Unbundle By Name(w4315) -> ("DO parameters"=w4314:T18)
                                n1678 = Index Array(array=w4314, index=w4313) -> (element=w4312:T19)
                                }
                                frame #1 {
                                w4326 = 0.0 ("padding value")
                                n1679 = call "2pparameters.vi"("command"="get") -> ("params out"=w4324:T11)  [unwired: 1 in]
                                n1680 = Unbundle By Name(w4324) -> ("srate"=w4321:sgl, "Pel"=w4323:sgl)
                                n1681 = To Double Precision Float(number=w4321) -> (double precision float=w4319:dbl)
                                n1682 = To Double Precision Float(number=w4321) -> (double precision float=w4320:dbl)
                                n1683 = To Double Precision Float(number=w4323) -> (double precision float=w4322:dbl)
                                n1684 = Divide(x=w4320, y=w4322) -> (x/y=w4318:dbl)
                                n1685 = call "replace DO wf param.vi"("Digital Freq (Hz)"=w4318, "Digital DC (%)"=100.0, "Digital phase"=w4326, "Sampling frequency (Hz)"=w4319, "Digital time offset (s)"=w4326, "index of DO wave"=w4327, "padding value"=w4326, "matlab wave file"=path "2Pshutter" ("matlab wave number")) -> ()  [unwired: 3 in]
                                }
                                }
                                }
                                frame True {
                                }
                                }
                                }
                                }
                                n1686 = Build Array(w4301) -> (w4300:T18)
                                }
                                }
                                }
                                frame #7 {
                                n1687 = Build Array(w4332, w4331) -> (w4334:bool[])
                                n1688 = Boolean Array To Number(Boolean array=w4334) -> (number=w4333:u32)
                                n1689 = case shown="0" w4333 {
                                tunnel: w4330 -> [_ w4376 _ w4383]
                                tunnel: [_ w4375 _ w4381] -> w4329
                                frame 1 {
                                n1690 = call "2pparameters.vi"("command"="get") -> ("params out"=w4341:T11)  [unwired: 1 in]
                                n1691 = Unbundle By Name(w4341) -> ("wavdet"=w4342:bool, "Pel"=w4344:sgl, "refwfsize"=w4345:dbl, "srateAODO"=w4343:sgl)
                                n1692 = call "waveformsDObuffer.vi"("command"="get") -> ("DO wf out"=w4337:digitalwaveform[])  [unwired: 1 in]
                                n1693 = case shown="False" w4342 {
                                tunnel: [w4350 w4360] -> w4339
                                tunnel: w4343 -> [w4355 w4371]
                                tunnel: w4344 -> [w4349 w4364]
                                tunnel: w4345 -> [_ w4368]
                                frame False {
                                w4353 = u16 0 items=["unsigned binary", "offset binary", "2's complement"] ("data format (offset binary)")
                                n1694 = Initialize Array(sgl 1.0, w4349) -> (w4346:sgl[])
                                n1695 = Reciprocal(x=w4355) -> (1/x=w4356:sgl)
                                n1696 = Bundle By Name("Y"=w4346, "dt"=w4356) -> (w4351:waveform(sgl))  [unwired: 1 in]
                                n1697 = call-poly <vilib>:"Analog to Digital.vi"("data format (offset binary)"=w4353, "compress digital (T)"=TRUE, "full-scale range (pk-pk)"=1.0, "resolution (16 bit)"=1, "analog waveform"=w4351) -> ("digital waveform"=w4350:digitalwaveform)  [unwired: 3 in, 3 out]
                                }
                                frame True {
                                w4363 = u16 0 items=["unsigned binary", "offset binary", "2's complement"] ("data format (offset binary)")
                                n1698 = To Double Precision Float(number=w4364) -> (double precision float=w4369:dbl)
                                n1699 = Initialize Array(sgl 1.0, w4364) -> (w4357:sgl[])
                                n1700 = Divide(x=w4368, y=w4369) -> (x/y=w4366:dbl)
                                n1701 = Round Toward +Infinity(x=w4366) -> (ceil(x): smallest int >= x=w4367:dbl)
                                n1702 = for {
                                N: w4367 -> [_]
                                tunnel: w4357 -> [w4373]
                                tunnel: [w4373] -> w4370 mode=concatenating
                                }
                                n1703 = Reciprocal(x=w4371) -> (1/x=w4372:sgl)
                                n1704 = Bundle By Name("Y"=w4370, "dt"=w4372) -> (w4361:waveform(sgl))  [unwired: 1 in]
                                n1705 = call-poly <vilib>:"Analog to Digital.vi"("data format (offset binary)"=w4363, "compress digital (T)"=TRUE, "full-scale range (pk-pk)"=1.0, "resolution (16 bit)"=1, "analog waveform"=w4361) -> ("digital waveform"=w4360:digitalwaveform)  [unwired: 3 in, 3 out]
                                }
                                }
                                n1706 = Build Array (concatenate)(w4337, w4339) -> (w4335:digitalwaveform[])
                                n1707 = call "waveformsDObuffer.vi"("DO wf in"=w4335, "command"="set") -> ()  [unwired: 1 out]
                                }
                                frame 2 {
                                n1708 = call "waveformsDObuffer.vi"("command"="get") -> ("DO wf out"=w4378:digitalwaveform[])  [unwired: 1 in]
                                n1709 = Delete From Array(array=w4378, length=1, index=w4376) -> (deleted portion=w4375:digitalwaveform[], array with subset deleted=w4374:digitalwaveform[])
                                n1710 = call "waveformsDObuffer.vi"("DO wf in"=w4374, "command"="set") -> ()  [unwired: 1 out]
                                }
                                frame 3, Default {
                                }
                                frame 0 {
                                n1711 = call "2pparameters.vi"("command"="get") -> ("params out"=w4385:T11)  [unwired: 1 in]
                                n1712 = Unbundle By Name(w4385) -> ("autoshutter"=w4384:bool, "wavdet"=w4382:bool)
                                n1713 = case shown="True" w4384 {
                                tunnel: w4383 -> [_ w4389]
                                tunnel: w4382 -> [_ w4388]
                                tunnel: [_ w4387] -> w4381
                                frame False {
                                }
                                frame True {
                                n1714 = case shown="False" w4388 {
                                tunnel: w4389 -> [w4393 _]
                                tunnel: [w4391 _] -> w4387
                                frame False {
                                w4400 = u16 0 items=["unsigned binary", "offset binary", "2's complement"] ("data format (offset binary)")
                                n1715 = call "2pparameters.vi"("command"="get") -> ("params out"=w4407:T11)  [unwired: 1 in]
                                n1716 = call "waveformsDObuffer.vi"("command"="get") -> ("DO wf out"=w4394:digitalwaveform[])  [unwired: 1 in]
                                n1717 = Unbundle By Name(w4407) -> ("Pel"=w4409:sgl, "srate"=w4408:sgl)
                                n1718 = Index Array(array=w4394, index=w4393) -> (element=w4392:digitalwaveform)
                                n1719 = Build Array(w4392) -> (w4391:digitalwaveform[])
                                n1720 = Initialize Array(sgl 1.0, w4409) -> (w4395:sgl[])
                                n1721 = Reciprocal(x=w4408) -> (1/x=w4402:sgl)
                                n1722 = Bundle By Name("Y"=w4395, "dt"=w4402) -> (w4398:waveform(sgl))  [unwired: 1 in]
                                n1723 = call-poly <vilib>:"Analog to Digital.vi"("data format (offset binary)"=w4400, "compress digital (T)"=TRUE, "full-scale range (pk-pk)"=1.0, "resolution (16 bit)"=1, "analog waveform"=w4398) -> ("digital waveform"=w4405:digitalwaveform)  [unwired: 3 in, 3 out]
                                n1724 = Replace Array Subset(array=w4394, new element=w4405, index=w4393) -> (w4390:digitalwaveform[])
                                n1725 = call "waveformsDObuffer.vi"("DO wf in"=w4390, "command"="set") -> ()  [unwired: 1 out]
                                }
                                frame True {
                                }
                                }
                                }
                                }
                                }
                                }
                                }
                                frame #8 {
                                n1726 = Build Array(w4413, w4412) -> (w4415:bool[])
                                n1727 = Boolean Array To Number(Boolean array=w4415) -> (number=w4414:u32)
                                n1728 = case shown="0" w4414 {
                                tunnel: w4411 -> [_ w4441 _ w4453]
                                tunnel: [_ w4440 _ w4451] -> w4410
                                frame 1 {
                                w4428 = 0.0 ("DOtab")
                                n1729 = call "2pparameters.vi"("command"="get") -> ("params out"=w4426:T11)  [unwired: 1 in]
                                n1730 = call "waveformparamsv2.vi"("command"="get") -> ("Params out"=w4436:T15)  [unwired: 4 in, 2 out]
